vi "PDC_Init.vi"(8 "error in (no error)":errorcluster) -> (0 "error out":errorcluster, 2 "ErrorCode":u32, 3 "ReturnValue":u32)   [LabVIEW 2015]
doc: "This VI initializes PDCLIB."
uses:
  PDCLIB.dll
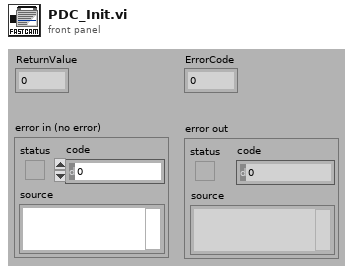
[diagram p1: front panel]
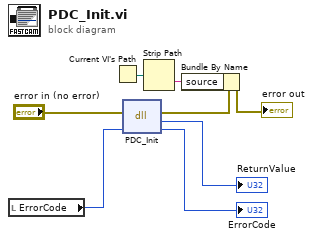
[diagram p0: block diagram]
diagram:
  n1 = local read "ErrorCode"() -> (w5:u32)
  n2 = Current VI's Path() -> (path=w3:path)
  n3 = dll-call lib="PDCLIB.dll" fn="PDC_Init"(error in="error in (no error)", "pErrorCode"=w5) -> (error out=w2:errorcluster, "return type"=→"ReturnValue":u32, "pErrorCode"=→"ErrorCode":u32)  [unwired: 2 in, 1 out]
  n4 = Strip Path(path=w3) -> (name=w4:string)  [unwired: 1 out]
  n5 = Bundle By Name(cluster=w2, "source"=w4) -> (→"error out":errorcluster)
